vi "Pack Errors.vi"(8 "Error In":errorcluster, 10 "Error Code":i32) -> (0 "Error Out":errorcluster)   [LabVIEW 2014, in "LQ Core.lvlib"]
uses:
  LQ Core.lvlib
panel:
  # "Copyright (c) 2016 Sze Howe Koh\n\nThis Source Code Form is subject to the terms of the Mozilla Public\nLicense, v. 2.0. If a copy of the MPL was not distributed with this\nfile, You can obtain one at http://mozilla.org/MPL/2.0/."
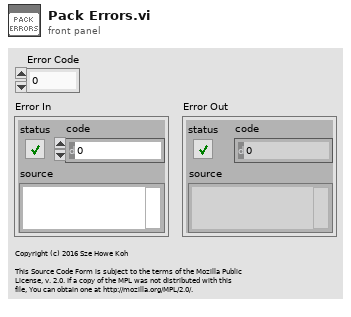
[diagram p1: front panel]
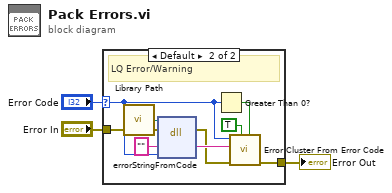
[diagram p0: block diagram]
diagram:
  n1 = case shown="Default" "Error Code" {
    selector: "Error Code" -> [_ w9]
    tunnel: "Error In" -> [w4 w6]
    tunnel: [w4 w13] -> w2
    frame 0 {
      # "No LQ-specific error/warning"
    }
    frame Default {
      # "LQ Error/Warning"
      n2 = call "Library Path.vi"() -> ("Library Path"=w10:path)
      n3 = dll-call lib="?" fn="errorStringFromCode"(path in=w10, error in=w6, "retVal"="", "errorCode"=w9) -> (error out=w5:errorcluster, "retVal"=w7:string)  [unwired: 3 in, 1 out]
      n4 = Greater Than 0?(x=w9) -> (x > 0?=w11:bool)
      n5 = call <vilib>:"Error Cluster From Error Code.vi"("is warning? (False)"=w11, "show call chain? (False)"=TRUE, "error in (no error)"=w5, "error message (\"\")"=w7, "error code (0)"=w9) -> ("error out"=w13:errorcluster)  [unwired: 4 in]
    }
  }
  "Error Out" <- w2
